vi "Read configuration.vi"(8 "error in (no error)":errorcluster, 11 "Switch Channel in":refnum<class "Switch Channel.lvclass">) -> (0 "error out":errorcluster, 2 "configuration":refnum<class "CEF_serializable configuration.lvclass">, 3 "Switch Channel out":refnum<class "Switch Channel.lvclass">)   [LabVIEW 2025, in "Switch.lvlib" / "Switch Channel.lvclass"]
uses:
  Switch Channel.lvclass
  Users/Public/Documents/Sandia National Labs/TSS Plugin/CEF.lvlibp/serializable configuration/CEF_serializable configuration.lvclass
  Switch Channel.lvclass/Switch Channel.ctl
  Switch configuration/Switch Channel configuration.lvclass
  Switch Channel configuration/Switch Channel configuration.lvclass
  C:/Users/Public/Documents/Sandia National Labs/TSS Plugin/Abstract PlugIn.lvlibp/Plugin/Abstract/Channel configuration/Channel configuration.lvclass
  C:/Users/Public/Documents/Sandia National Labs/TSS Plugin/CEF.lvlibp/serializable configuration/CEF_serializable configuration.lvclass
  C:/Working copy/tss/Plugin/Engines/Switch/Switch Channel configuration/Switch Channel configuration.lvclass
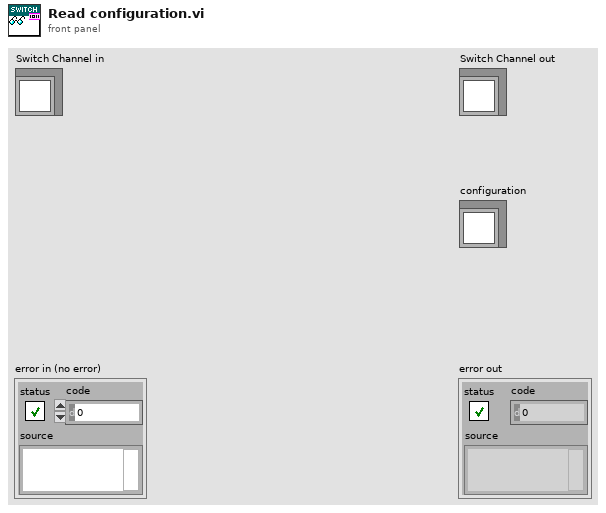
[diagram p1: front panel]
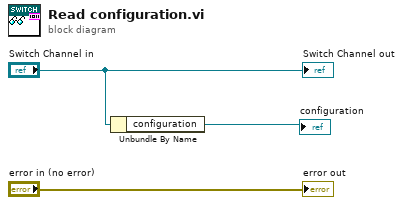
[diagram p0: block diagram]
diagram:
  n1 = Unbundle By Name("Switch Channel in") -> ("configuration"=→"configuration":refnum<class "Switch Channel configuration.lvclass">)
  "error out" <- "error in (no error)"
  "Switch Channel out" <- "Switch Channel in"
